vi "AWG Send Script Trigger.vi"(7 "trigger id (script trigger 0)":T1="ScriptTrigger0", 8 "error in (no error)":errorcluster, 10 "Delay Time (s)":dbl, 11 "AWG Sessions In":refnum<k15>[](array[refnum])) -> (0 "error out":errorcluster, 3 "AWG Sessions Out":refnum<k15>[](array[refnum]))   [LabVIEW 2013]
doc: "Sends the selected script trigger for HSDIO sessions"
uses:
  <instrlib>/niHSDIO/niHSDIO.llb/niHSDIO_ctl Trigger Script - trigID Values (Ring).ctl
  <instrlib>/niFgen/niFgen.llb/niFgen_ctl Trigger SW - TrigName Values (Ring).ctl
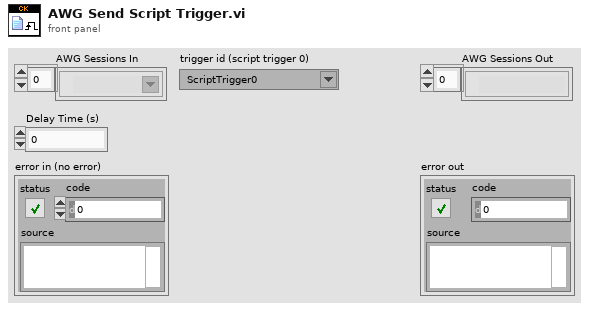
[diagram p1: front panel]
types:
  T1 = typedef "niHSDIO_ctl Trigger Script - trigID Values (Ring).ctl" = string
  T2 = typedef "niFgen_ctl Trigger SW - TrigName Values (Ring).ctl" = i32
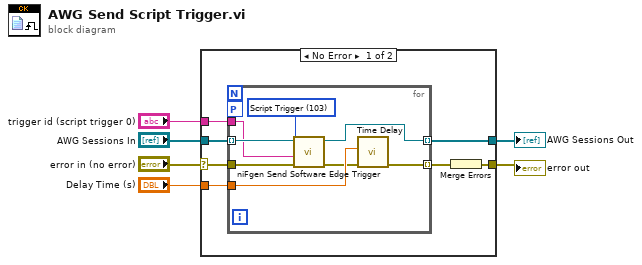
[diagram p0: block diagram]
diagram:
  n1 = case shown="No Error" "error in (no error)" {
    selector: "error in (no error)" -> [w7 w23]
    tunnel: [w13 w23] -> w6
    tunnel: "AWG Sessions In" -> [w12 w22]
    tunnel: "trigger id (script trigger 0)" -> [w11 _]
    tunnel: [w9 w22] -> w3
    tunnel: "Delay Time (s)" -> [w8 _]
    frame No Error {
      n2 = for {
        tunnel: w12 -> [w17] mode=indexing
        tunnel: w7 -> [w15]
        tunnel: w11 -> [w16]
        tunnel: [w21] -> w10 mode=indexing
        tunnel: [w18] -> w9 mode=indexing
        tunnel: w8 -> [w20]
        workers-P: _ -> [_]
        w14 = T2 103 items=["Start Trigger"=1004, "Script Trigger"=103] ("Trigger (Start Trigger)")
        n3 = call <instrlib>:"niFgen Send Software Edge Trigger.vi"("error in (no error)"=w15, "Trigger ID (None)"=w16, "Trigger (Start Trigger)"=w14, "Instrument Handle"=w17) -> ("error out"=w19:errorcluster, "Instrument Handle Out"=w18:refnum<k15>)  [unwired: 6 in]
        n4 = call "Time Delay"("error in (no error)"=w19, "Delay Time (s)"=w20) -> ("error out"=w21:errorcluster)  [unwired: 9 in]
      }
      n5 = Merge Errors(w10) -> (w13:errorcluster)
    }
    frame Error {
    }
  }
  "AWG Sessions Out" <- w3
  "error out" <- w6
